vi "Get Row and Column.vi"(0 "Component in":refnum<class "Component.lvclass">) -> (1 "row":i16, 2 "column":i16)   [LabVIEW 2023, in "Component.lvclass"]
doc: "Get this component's position."
uses:
  Component.lvclass
  Component.lvclass/Component.ctl
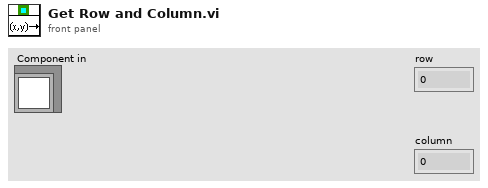
[diagram p1: front panel]
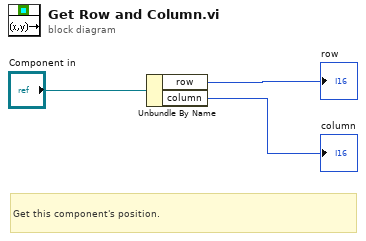
[diagram p0: block diagram]
diagram:
  # "Get this component's position."
  n1 = Unbundle By Name("Component in") -> ("row"=→"row":i16, "column"=→"column":i16)
